vi "Generate AO Sample Clock.vi"() -> ()   [LabVIEW 2010]
doc: "I. Description:\nThis example generates a clock of variable rate for the analog output circuitry. An array of 0V is the actual output, so the example is merely used to generate an analog clock.\n\nII. Instructions for Running:\n1. Select the Physical Channel to correspond to where an analog output channel on the DAQ device.\n2. Specify the desired Output Clock Rate (Hz). This control can be modified while the generation is taking place."
uses:
  <vilib>/DAQmx/write.llb/DAQmx Write (Analog 1D DBL 1Chan NSamp).vi
  <vilib>/DAQmx/create/channels.llb/DAQmx Create Channel (AO-Voltage-Basic).vi
  <vilib>/DAQmx/configure/timing.llb/DAQmx Timing (Sample Clock).vi
  <vilib>/daqmx/miscellaneous.llb/DAQmx Fill In Error Info.vi
  ni/labview/resource/objmgr/daqmx.rc
panel:
  in  "Output Clock Rate (Hz)":dbl(slide)=1000.0 caption="Desired Frequency" scale=1.0..100.0
  in  "Physical Channels":tag="Dev1/ao0:1"
  in  "stop":bool
  # "Channel Parameters"
  # "Timing Parameters"
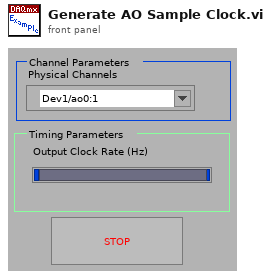
[diagram p1: front panel]
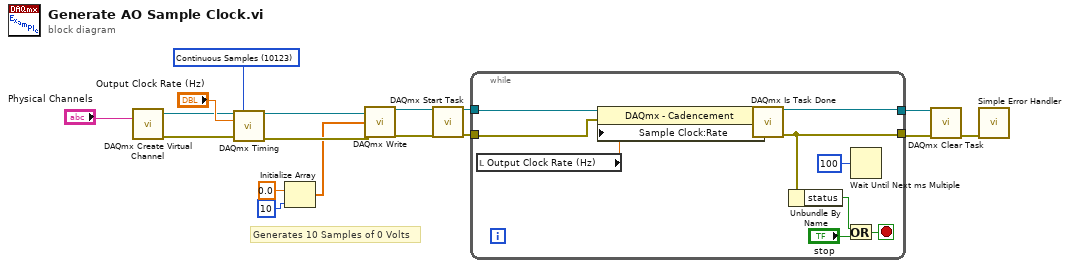
[diagram p0: block diagram]
diagram:
  w16 = 10123 items=["Finite Samples"=10178, "Continuous Samples"=10123] ("sample mode")
  # "Generates 10 Samples of 0 Volts"
  n1 = call-poly <vilib>:"DAQmx Create Virtual Channel.vi"("physical channels"="Physical Channels") -> ("task out"=w2:refnum<k21>, "error out"=w1:errorcluster)  [unwired: 13 in]
  n2 = call-poly <vilib>:"DAQmx Timing.vi"("task/channels in"=w2, "sample mode"=w16, "rate"="Output Clock Rate (Hz)", "error in"=w1) -> ("task out"=w11:refnum<k21>, "error out"=w7:errorcluster)  [unwired: 10 in]
  n3 = Initialize Array(0.0 ("element"), 10 ("dimension size")) -> (w3:dbl[])
  n4 = call-poly <vilib>:"DAQmx Write.vi"("task/channels in"=w11, "data"=w3, "error in"=w7) -> ("task out"=w15:refnum<k21>, "error out"=w14:errorcluster)  [unwired: 10 in, 1 out]
  n5 = call <vilib>:"DAQmx Start Task.vi"("task/channels in"=w15, "error in"=w14) -> ("task out"=w17:refnum<k21>, "error out"=w13:errorcluster)  [unwired: 12 in]
  n6 = while {
    tunnel: w17 -> [w20]
    tunnel: [w23] -> w9
    tunnel: w13 -> [w19]
    tunnel: [w24] -> w8
    stop <- w28 stop-if-true
    n7 = local read "Output Clock Rate (Hz)"() -> (w18:dbl)
    n8 = property class="DAQmx - Cadencement"(reference=w20, error in=w19, "Sample Clock:Rate"=w18) -> (reference out=w22:refnum<k21>, error out=w21:errorcluster)
    n9 = call <vilib>:"DAQmx Is Task Done.vi"("task/channels in"=w22, "error in"=w21) -> ("task out"=w23:refnum<k21>, "error out"=w24:errorcluster)  [unwired: 11 in, 1 out]
    n10 = Unbundle By Name(w24) -> ("status"=w26:bool)
    n11 = Or(x=w26, y="stop") -> (x .or. y?=w28:bool)
    n12 = Wait Until Next ms Multiple(millisecond multiple=u32 100) -> ()  [unwired: 1 out]
  }
  n13 = call <vilib>:"DAQmx Clear Task.vi"("task in"=w9, "error in"=w8) -> ("error out"=w10:errorcluster)  [unwired: 13 in]
  n14 = call <vilib>:"Simple Error Handler.vi"("error in (no error)"=w10) -> ()  [unwired: 4 in, 5 out]
